vi "cdf.vi"(11 "Array":dbl[](array[numeric])) -> (3 "Cluster":cluster{dbl[], dbl[]})   [LabVIEW 2020]
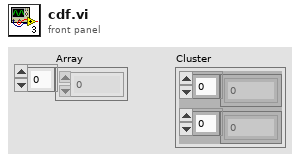
[diagram p1: front panel]
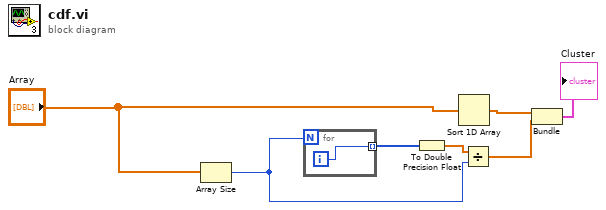
[diagram p0: block diagram]
diagram:
  n1 = Array Size(array="Array") -> (size(s)=w2:i32)
  n2 = for {
    N: w2 -> [_]
    tunnel: [w8] -> w4 mode=indexing
    i -> [w8]
  }
  n3 = To Double Precision Float(number=w4) -> (double precision float=w3:dbl[])
  n4 = Sort 1D Array(array="Array") -> (sorted array=w5:dbl[])
  n5 = Divide(x=w3, y=w2) -> (x/y=w1:dbl[])
  n6 = Bundle(w5, w1) -> (→"Cluster":cluster{dbl[], dbl[]})  [unwired: 1 in]
